vi "Utility_Get Colors and Count 1D Array.vi"(8 "Error":errorcluster, 11 "Color Array":u32[](array[colorbox])) -> (0 "Error Out":errorcluster, 2 "Count Out":u32[](array[numeric]), 3 "Color List Out":u32[](array[colorbox]))   [LabVIEW 2009]
doc: "Seperates a color array into the colors array and the color count array"
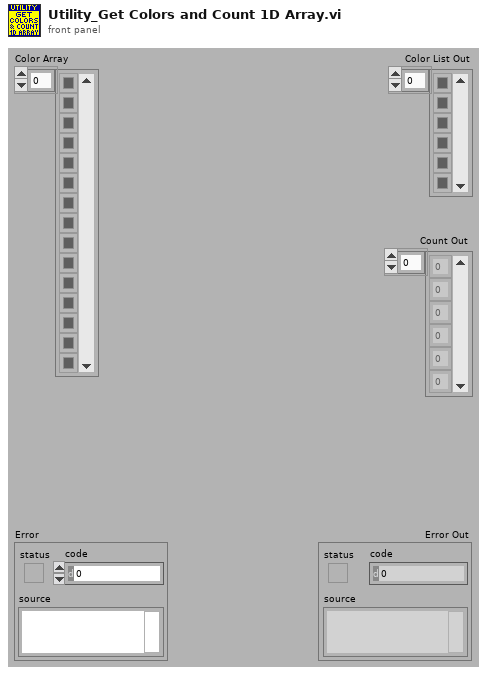
[diagram p1: front panel]
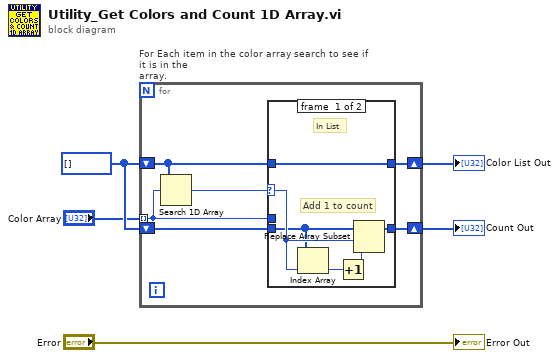
[diagram p0: block diagram]
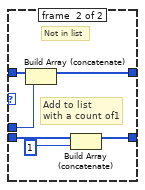
[diagram p2: hidden frame]
diagram:
  w4 = u32[] [] ("colors")
  n1 = for "For Each item in the color array search to see if it is in the\narray." {
    tunnel: "Color Array" -> [w8] mode=indexing
    shift-right: [w11] -> w2
    shift-left: w4 -> [w10]
    shift-right: [w6] -> w5
    shift-left: w4 -> [w7]
    n2 = Search 1D Array(1D array=w10, element=w8) -> (index of element=w9:i32)  [unwired: 1 in]
    n3 = case shown="0, Default" w9 {
      selector: w9 -> [w14 _]
      tunnel: w10 -> [w17 w23]
      tunnel: [w17 w22] -> w11
      tunnel: w8 -> [_ w21]
      tunnel: w7 -> [w13 w20]
      tunnel: [w12 w19] -> w6
      frame #0 {
        # "Add 1 to count"
        # "In List"
        n4 = Index Array(array=w13, index=w14) -> (element=w16:u32)
        n5 = Increment(x=w16) -> (x+1=w15:u32)
        n6 = Replace Array Subset(array=w13, new element=w15, index=w14) -> (w12:u32[])
      }
      frame #1 {
        # "Add to list\nwith a count of1"
        # "Not in list"
        n7 = Build Array (concatenate)(w23, w21) -> (w22:u32[])
        n8 = Build Array (concatenate)(w20, u32 1) -> (w19:u32[])
      }
    }
  }
  "Count Out" <- w5
  "Color List Out" <- w2
  "Error Out" <- "Error"
